vi "Add Directory to Tree View.vi"(1 "Show Full Directory Path ? (F)":bool, 2 "Directory Tree in":T1, 3 "Item Indent":i32, 4 "Directory":string) -> (0 "Tree View":T4(array[cluster]))   [LabVIEW 2020, in "AoC 2022.lvlib"]
uses:
  AoC 2022.lvlib
  Directory Tree.ctl
  Directory Contents.ctl
  File.ctl
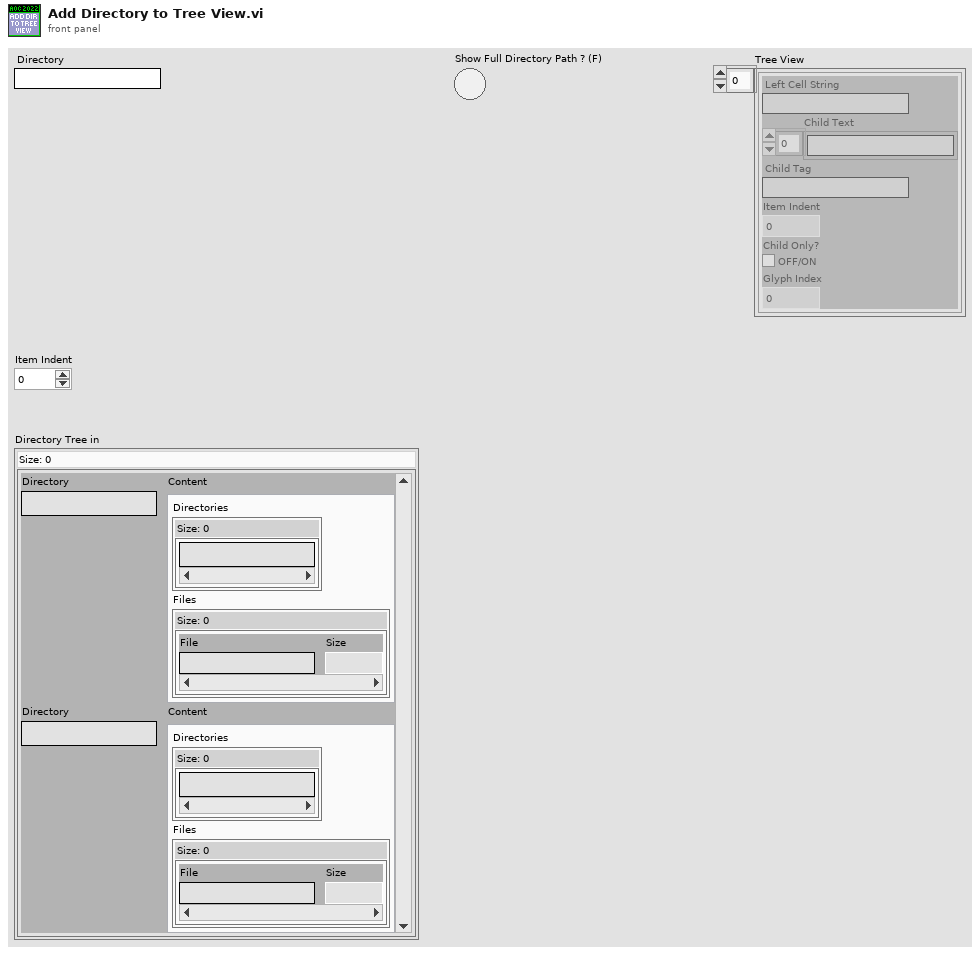
[diagram p1: front panel]
types:
  T1 = typedef "AoC 2022.lvlib/Directory Tree.ctl" = map{string, T2}
  T2 = typedef "AoC 2022.lvlib/Directory Contents.ctl" = cluster{"Directories":set{string}, "Files":T3}
  T3 = typedef "AoC 2022.lvlib/File.ctl" = map{string, u64}
  T4 = cluster{"Left Cell String":string, "Child Text":string[], "Child Tag":string, "Item Indent":i32, "Child Only?":bool, "Glyph Index":i32}[]
  T5 = cluster{"Left Cell String":string, "Child Text":string[], "Child Tag":string, "Item Indent":i32, "Child Only?":bool, "Glyph Index":i32}
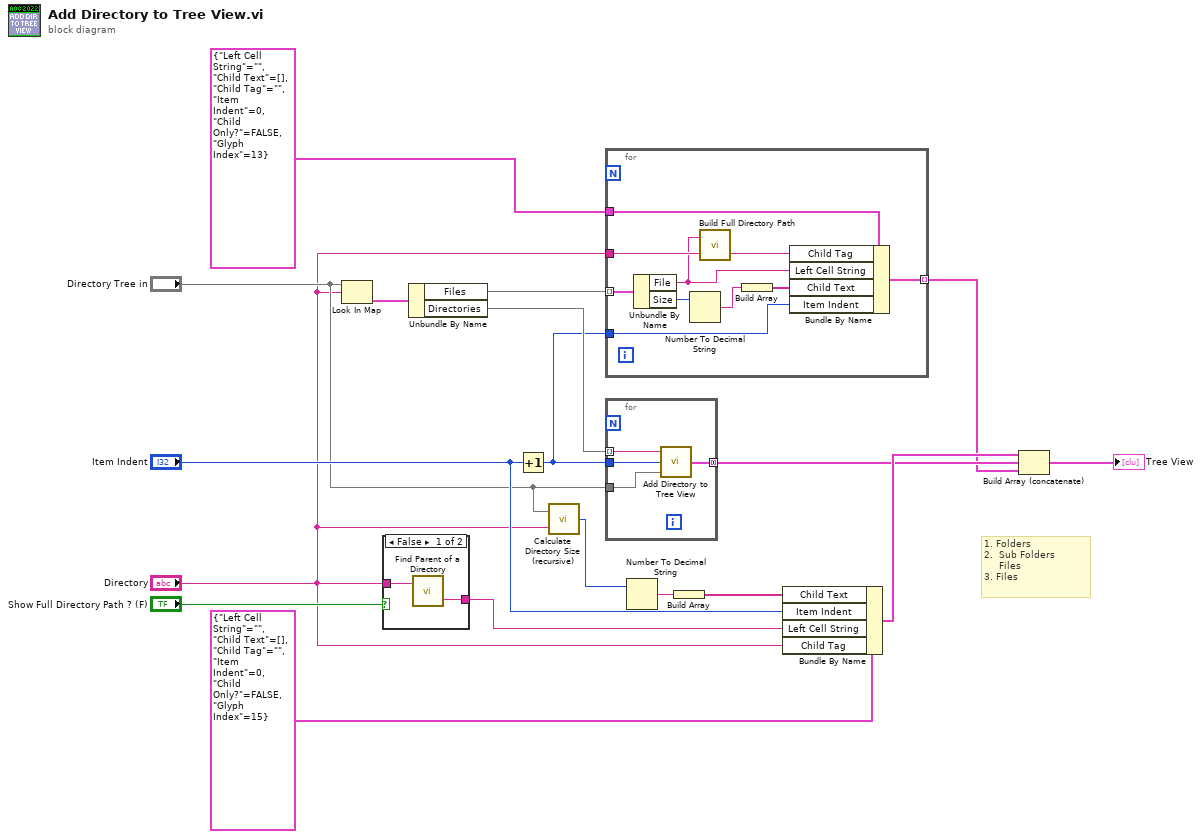
[diagram p0: block diagram]
diagram:
  # "1. Folders\n2.  Sub Folders\n     Files\n3. Files"
  n1 = Look In Map(map="Directory Tree in", key="Directory") -> (value=w11:T2)  [unwired: 1 in, 1 out]
  n2 = case shown="False" "Show Full Directory Path ? (F)" {
    tunnel: [w20 w21] -> w16
    tunnel: "Directory" -> [w19 w21]
    frame False {
      n3 = call "Find Parent of a Directory.vi"("Directory"=w19) -> ("Directory (stripped)"=w20:string)  [unwired: 1 in, 1 out]
    }
    frame True {
    }
  }
  n4 = Unbundle By Name(w11) -> ("Files"=w12:T3, "Directories"=w14:set{string})
  n5 = Increment(x="Item Indent") -> (x+1=w1:i32)
  n6 = call "Calculate Directory Size (recursive).vi"("Directory"="Directory", "Directory Tree"="Directory Tree in") -> ("Directory Size"=w4:u64)
  n7 = for {
    tunnel: w12 -> [w29] mode=indexing
    tunnel: T5 {"Left Cell String"="", "Child Text"=[], "Child Tag"="", "Item Indent"=0, "Child Only?"=FALSE, "Glyph Index"=13} ("Item") -> [w31]
    tunnel: w1 -> [w30]
    tunnel: "Directory" -> [w28]
    tunnel: [w22] -> w8 mode=indexing
    n8 = Unbundle By Name(w29) -> ("File"=w26:string, "Size"=w25:u64)
    n9 = Number To Decimal String(number=w25) -> (decimal integer string=w24:string)  [unwired: 1 in]
    n10 = call "Build Full Directory Path.vi"("Parent Directory"=w28, "Sub Directory"=w26) -> ("Full Directory Path"=w27:string)  [unwired: 1 in]
    n11 = Build Array(w24) -> (w23:string[])
    n12 = Bundle By Name(cluster=w31, "Child Tag"=w27, "Left Cell String"=w26, "Child Text"=w23, "Item Indent"=w30) -> (w22:T5)
  }
  n13 = for {
    tunnel: w14 -> [w33] mode=indexing
    tunnel: [w35] -> w9 mode=concatenating
    tunnel: w1 -> [w34]
    tunnel: "Directory Tree in" -> [w32]
    n14 = call "Add Directory to Tree View.vi"("Directory Tree in"=w32, "Item Indent"=w34, "Directory"=w33) -> ("Tree View"=w35:T4)  [unwired: 1 in]
  }
  n15 = Number To Decimal String(number=w4) -> (decimal integer string=w3:string)  [unwired: 1 in]
  n16 = Build Array(w3) -> (w2:string[])
  n17 = Bundle By Name(cluster=T5 {"Left Cell String"="", "Child Text"=[], "Child Tag"="", "Item Indent"=0, "Child Only?"=FALSE, "Glyph Index"=15} ("Item"), "Child Text"=w2, "Item Indent"="Item Indent", "Left Cell String"=w16, "Child Tag"="Directory") -> (w10:T5)
  n18 = Build Array (concatenate)(w10, w9, w8) -> (→"Tree View":T4)
